vi "Get Combine Data.vi"(8 "error in (no error)":errorcluster, 11 "Scan Data Process in":T1) -> (0 "error out":errorcluster, 3 "Scan Data Process out":T1)   [LabVIEW 2015, in "Exposure Process.lvlib"]
uses:
  Exposure Process.lvlib
  Control_Scan Data Process.ctl
  <vilib>/addons/PointValueMap/controls/PointMap.ctl
  Control_EXP Information.ctl
  Control_File Save Setup.ctl
  Control_Enable and Path.ctl
  Control_ICM Export Setting.ctl
  <vilib>/addons/PointValueMap/PointValueMap.lvlib
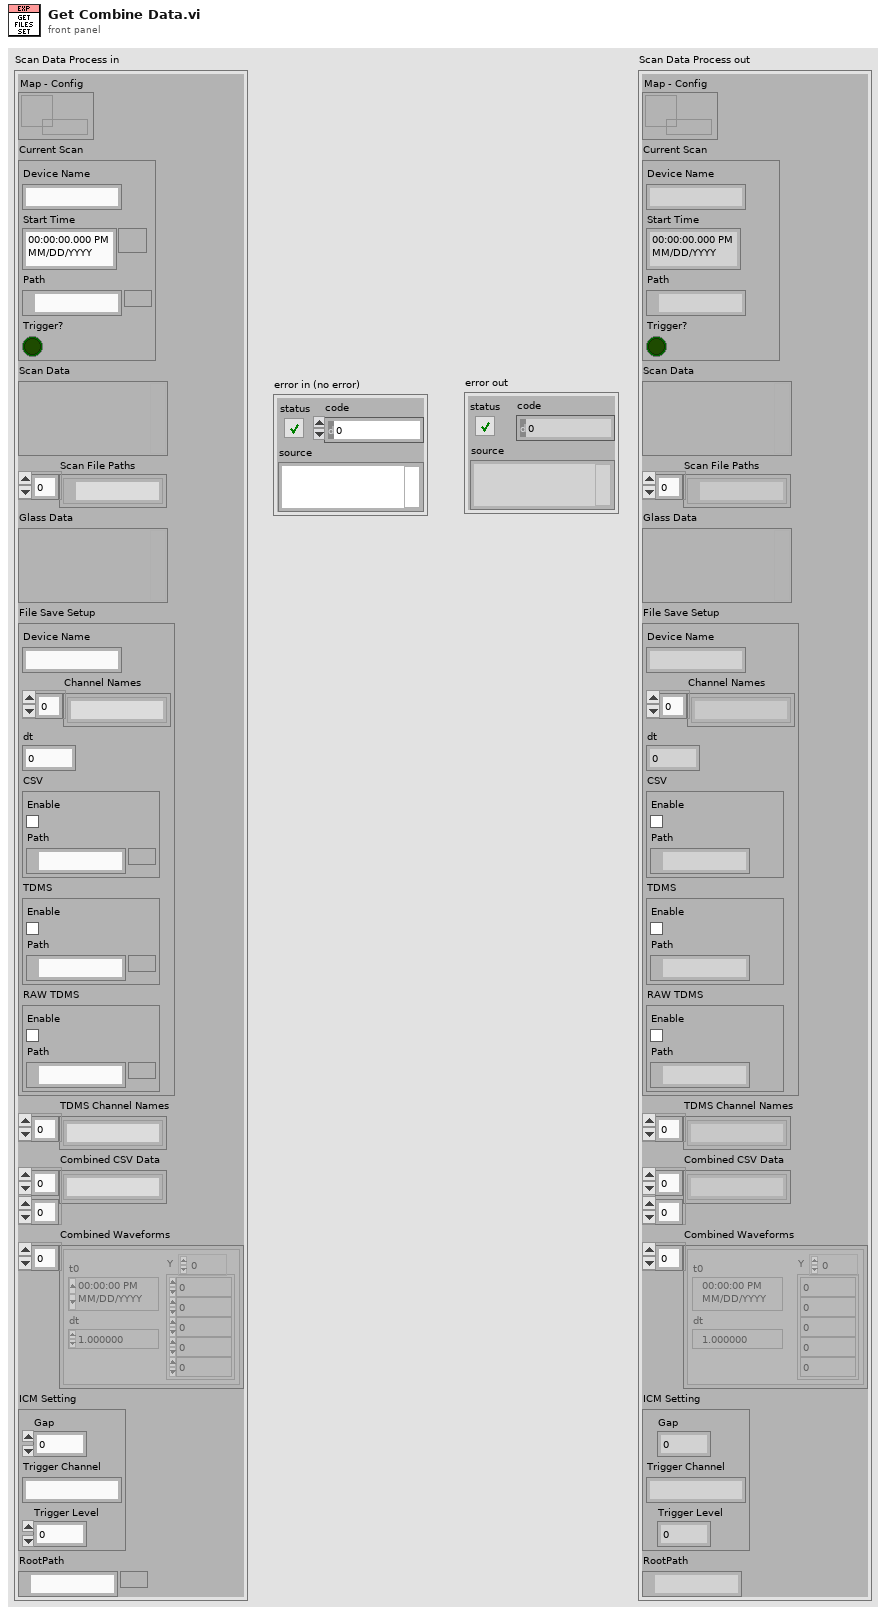
[diagram p1: front panel]
types:
  T1 = typedef "Exposure Process.lvlib/Control_Scan Data Process.ctl" = cluster{"Map - Config":T2, "Current Scan":T3, "Scan Data":variant, "Scan File Paths":path[], "Glass Data":variant, "File Save Setup":T4, "TDMS Channel Names":string[], "Combined CSV Data":string[][], "Combined Waveforms":waveform(dbl)[], "ICM Setting":T6, "RootPath":path}
  T2 = typedef "PointValueMap.lvlib/PointMap.ctl" = refnum<data-value>
  T3 = typedef "Exposure Process.lvlib/Control_EXP Information.ctl" = cluster{"Device Name":string, "Start Time":timestamp, "Path":path, "Trigger?":bool}
  T4 = typedef "Exposure Process.lvlib/Control_File Save Setup.ctl" = cluster{"Device Name":string, "Channel Names":string[], "dt":dbl, "CSV":T5, "TDMS":T5, "RAW TDMS":T5}
  T5 = typedef "Exposure Process.lvlib/Control_Enable and Path.ctl" = cluster{"Enable":bool, "Path":path}
  T6 = typedef "Exposure Process.lvlib/Control_ICM Export Setting.ctl" = cluster{"Gap":dbl, "Trigger Channel":string, "Trigger Level":dbl}
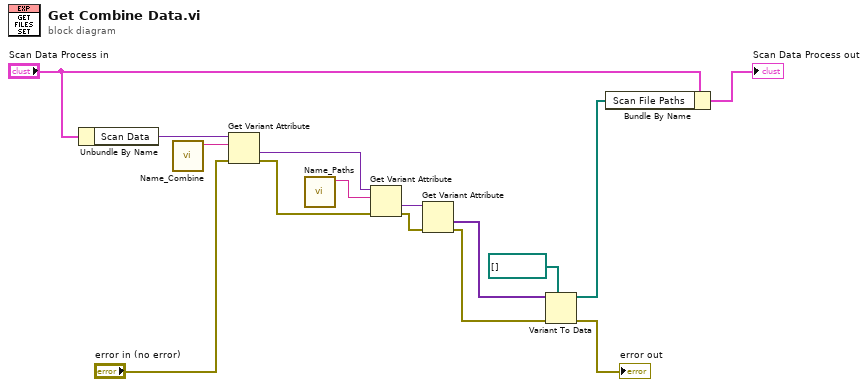
[diagram p0: block diagram]
diagram:
  n1 = Unbundle By Name("Scan Data Process in") -> ("Scan Data"=w9:variant)
  n2 = call "Name_Combine.vi"() -> ("Name"=w15:string)  [unwired: 11 in]
  n3 = Get Variant Attribute(Variant=w9, name=w15, error in="error in (no error)") -> (value=w14:variant, error out=w8:errorcluster)  [unwired: 1 in, 2 out]
  n4 = call "Name_Paths.vi"() -> ("Name"=w13:string)  [unwired: 11 in]
  n5 = Get Variant Attribute(Variant=w14, name=w13, error in=w8) -> (value=w12:variant, error out=w7:errorcluster)  [unwired: 1 in, 2 out]
  n6 = Get Variant Attribute(Variant=w12, error in=w7) -> (values=w11:variant[], error out=w6:errorcluster)  [unwired: 2 in, 2 out]
  n7 = Variant To Data(error in=w6, type=path[] [], Variant=w11) -> (data=w3:path[], error out=→"error out":errorcluster)
  n8 = Bundle By Name(cluster="Scan Data Process in", "Scan File Paths"=w3) -> (→"Scan Data Process out":T1)
